vi "Add - Core.vi"(0 "Error Filter in":refnum<class "Error Filter.lvclass">, 5 "Error Code":i32, 7 "Repetitions":u32, 9 "Time (s)":dbl, 11 "error in (no error)":errorcluster) -> (4 "Error Filter out":refnum<class "Error Filter.lvclass">, 15 "error out":errorcluster)   [LabVIEW 2026, in "TALOS.lvlib" / "Classes.lvlib" / "Error Filter.lvclass"]
doc: "Use this VI to add an error to be skipped in the future. If repetitions and time are both left to zero, the error will be permanently skipped: otherwise the error will be skipped until one of the two conditions will be met."
uses:
  Error Filter.lvclass
  Error Filter.lvclass/Error Filter.ctl
  Error Filter Properties.ctl
  <vilib>/Utility/miscctls.llb/LVMapReplaceAction.ctl
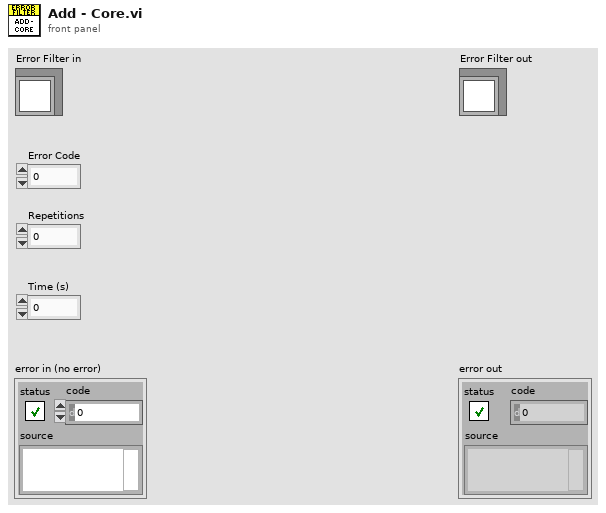
[diagram p1: front panel]
types:
  T1 = typedef "TALOS.lvlib/Classes.lvlib/Error Filter.lvclass/Error Filter Properties.ctl" = cluster{"Repetitions":u32, "Until":timestamp}
  T2 = typedef "LVMapReplaceAction.ctl" = enum32{"Modify Entry only if found", "Add or Modify Entry", "Delete Entry"}
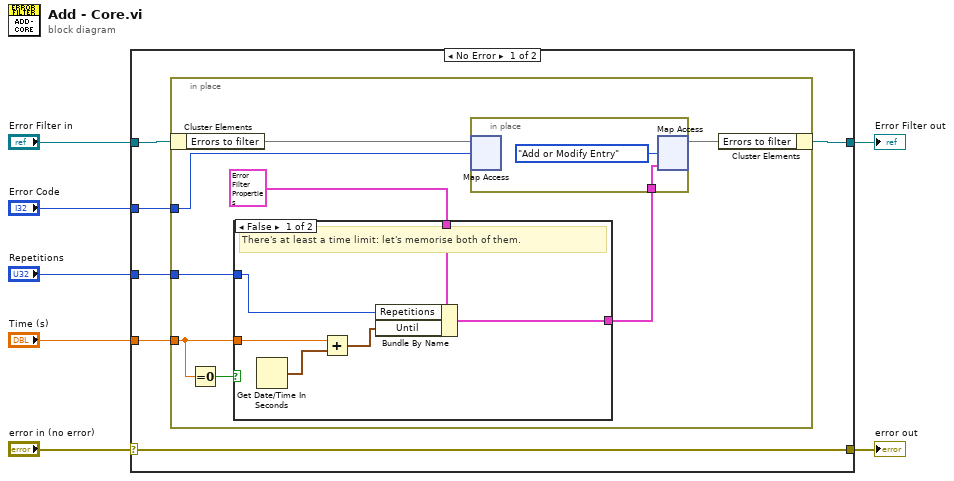
[diagram p0: block diagram]
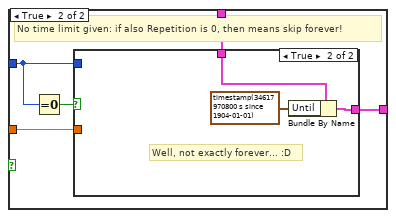
[diagram p2: hidden frame]
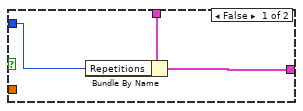
[diagram p3: hidden frame]
diagram:
  n1 = case shown="No Error" "error in (no error)" {
    selector: "error in (no error)" -> [w8 w42]
    tunnel: [w8 w42] -> w6
    tunnel: [w11 w41] -> w4
    tunnel: "Error Filter in" -> [w13 w41]
    tunnel: "Error Code" -> [w12 _]
    tunnel: "Repetitions" -> [w10 _]
    tunnel: "Time (s)" -> [w9 _]
    frame No Error {
      n2 = in-place {
        in-place-border: w12 -> [w20]
        in-place-border: w10 -> [w17]
        in-place-border: w9 -> [w15]
        n3 = in-place-cluster #1(w13) -> ("Errors to filter"=w21:map{i32, T1})
        n4 = Equal To 0?(x=w15) -> (x = 0?=w18:bool)
        n5 = case shown="False" w18 {
          tunnel: w17 -> [w23 w31]
          tunnel: T1 {"Repetitions"=1, "Until"=timestamp(0 s since 1904-01-01)} ("Error Filter Properties") -> [w27 w29]
          tunnel: w15 -> [w26 w30]
          tunnel: [w22 w28] -> w14
          frame False {
            # "There's at least a time limit: let's memorise both of them."
            n6 = Get Date/Time In Seconds() -> (seconds since 1Jan1904=w25:timestamp)
            n7 = Add(x=w26, y=w25) -> (x+y=w24:timestamp)
            n8 = Bundle By Name(cluster=w27, "Repetitions"=w23, "Until"=w24) -> (w22:T1)
          }
          frame True {
            # "No time limit given: if also Repetition is 0, then means skip forever!"
            n9 = Equal To 0?(x=w31) -> (x = 0?=w32:bool)
            n10 = case shown="True" w32 {
              tunnel: w31 -> [w34 _]
              tunnel: w30 -> [_ _]
              tunnel: w29 -> [w35 w38]
              tunnel: [w33 w37] -> w28
              frame False {
                n11 = Bundle By Name(cluster=w35, "Repetitions"=w34) -> (w33:T1)
              }
              frame True {
                # "Well, not exactly forever... :D"
                n12 = Bundle By Name(cluster=w38, "Until"=timestamp(34617970800 s since 1904-01-01)) -> (w37:T1)
              }
            }
          }
        }
        n13 = in-place {
          in-place-border: w14 -> [w39]
          n14 = in-place-map #2(w21, w20) -> ()  [unwired: 1 in, 2 out]
          n15 = in-place-map #2(w39, LVMapReplaceAction."Add or Modify Entry" ("action")) -> (w19:map{i32, T1})  [unwired: 2 out]
        }
        n16 = in-place-cluster #1("Errors to filter"=w19) -> (w11:refnum<class "Error Filter.lvclass">)
      }
    }
    frame Error {
    }
  }
  "error out" <- w6
  "Error Filter out" <- w4
